vi "Check Relationship of VI to Library.vi"(4 "Error In":errorcluster, 5 "Qualified Library Name":string, 6 "App Ref":refnum<vi>, 7 "VI Ref":refnum<vi>) -> (0 "Error Out":errorcluster, 1 "Relationship":T1, 2 "dup App Ref":refnum<vi>, 3 "dup VI Ref":refnum<vi>)   [LabVIEW 2025, in "XNode Support.lvlib"]
uses:
  XNode Support.lvlib
  Relationship of VI to Library.ctl
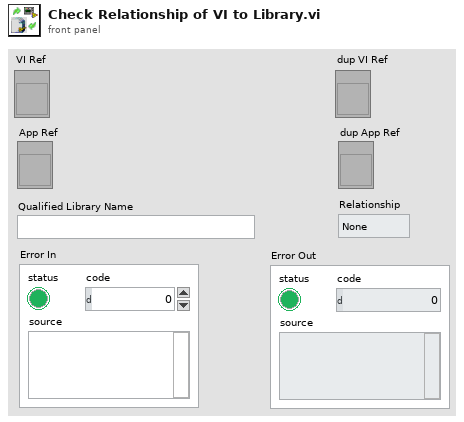
[diagram p1: front panel]
types:
  T1 = typedef "XNode Support.lvlib/Relationship of VI to Library.ctl" = enum16{"None", "Friend", "Member"}
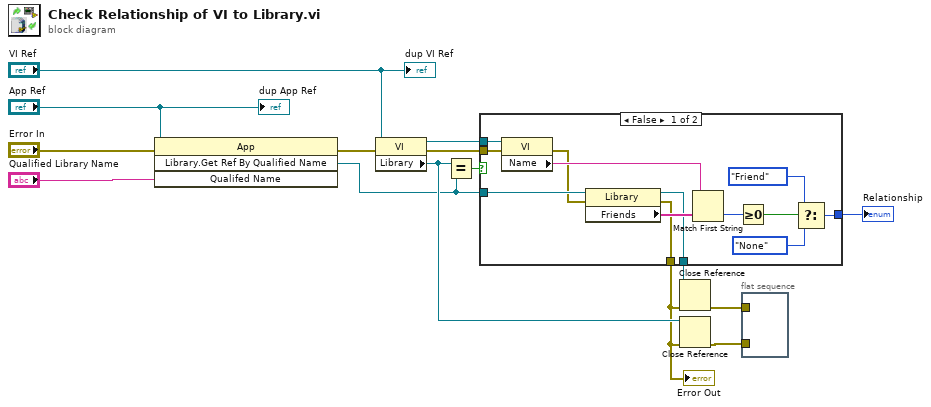
[diagram p0: block diagram]
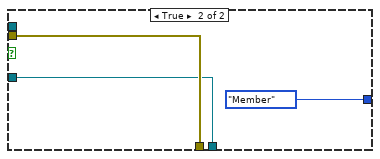
[diagram p2: hidden frame]
diagram:
  n1 = invoke class="App" method="Library.Get Ref By Qualified Name"(reference="App Ref", error in="Error In", "Qualifed Name"="Qualified Library Name") -> (error out=w9:errorcluster, "Library.Get Ref By Qualified Name"=w5:refnum<vi>)  [unwired: 1 in, 2 out]
  n2 = property class="VI"(reference="VI Ref", error in=w9) -> (reference out=w13:refnum<vi>, error out=w12:errorcluster, "Library"=w6:refnum<vi>)
  n3 = Equal?(x=w6, y=w5) -> (x = y?=w15:bool)
  n4 = case shown="False" w15 {
    tunnel: w5 -> [w28 w29]
    tunnel: [w20 Relationship_of_VI_to_Library."Member" ("Enum")] -> w14
    tunnel: w13 -> [w27 _]
    tunnel: w12 -> [w19 w30]
    tunnel: [w17 w30] -> w3
    tunnel: [w16 w29] -> w4
    frame False {
      n5 = property class="VI"(reference=w27, error in=w19) -> (error out=w18:errorcluster, "Name"=w25:string)  [unwired: 1 out]
      n6 = property class="Library"(reference=w28, error in=w18) -> (reference out=w16:refnum<vi>, error out=w17:errorcluster, "Friends"=w26:string[])
      n7 = Match First String(2:w26, 3:w25) -> (0:w24:i32)  [unwired: 1 out]
      n8 = Greater Or Equal To 0?(x=w24) -> (x >= 0?=w23:bool)
      n9 = Select(t=Relationship_of_VI_to_Library."Friend" ("Enum"), s=w23, f=Relationship_of_VI_to_Library."None" ("Enum")) -> (s? t:f=w20:T1)
    }
    frame True {
    }
  }
  "Relationship" <- w14
  "Error Out" <- w3
  n10 = Close Reference(reference=w4, error in (no error)=w3) -> (error out=w2:errorcluster)
  n11 = Close Reference(reference=w6, error in (no error)=w3) -> (error out=w1:errorcluster)
  n12 = flat-sequence {
    tunnel: w2 -> [_]
    tunnel: w1 -> [_]
    frame #0 {
    }
  }
  "dup App Ref" <- "App Ref"
  "dup VI Ref" <- "VI Ref"
